vi "Nicmos_Test.vi"() -> ()   [LabVIEW 2009]
uses:
  Controls/NICMOS.READOUT.ctl
  <vilib>/Analysis/2dsp.llb/Power Spectrum (DBL).vi
  <vilib>/Analysis/NI_AALBase.lvlib
  <vilib>/Analysis/NI_AALPro.lvlib
panel:
  in  "READOUT":T1={"Readout"=8, "Deglitch"=2, "Framerate"=40.061293779482604, "Bank"=6}
  in  "Commande onglet":T2(tab)=enum."Zoom"
  out "Std Dev 2":dbl=47.642857142857146 format="%.1f"
  out "Std Dev":dbl=6.902380541730306 format="%.1f"
  in  "Integrate pattern":bool
  out "Mean Level":dbl=112.25 format="%.1f"
  out "Total NRJ":i32=11694532
  out "Scan":i32[](graph)=[115, 117, 121, 110, 109, 113, 115, 98]
  out "Image":i32[][](graph)
  out "Power Spectrum":cluster{dbl[unit][], "Power Spectrum":dbl[]}(graph)={[0.0, 5.7230419684975145, 11.446083936995029, 17.169125905492542, 22.892167873990058, 28.615209842487573, 34.338251810985085, 40.0612937794826], "Power Spectrum"=[12600.0625, 4.685660171779821, 9.8125, 2.5643398282201786, 7.5625, 2.5643398282201786, 9.8125, 4.685660171779821]}
  out "y":dbl=39.77045768581225 format="%.1f"
  out "x":dbl=48.747249279268516 format="%.1f"
  out "b":dbl=0.5346203674875701 format="%.2f"
  out "theta":dbl[unit]=0.3638978669091496 format="%.2f"
  out "a":dbl=0.46263779966875623 format="%.2f"
  out "Graphe d'intensité 2":i32[][](graph)
  out "Y":dbl=40.58244294659929 format="%.2f"
  out "X":dbl=36.54206833038434 format="%.2f"
  out "Waist  Y":dbl=7.63982963428037 format="%.2f"
  out "Waist  X":dbl=1.8793090656266391 format="%.2f"
  out "Cut X":i32[](graph)=[103, 83, 96, 100, 88, 113, 103, 107, 94, 113, 101, 105, 126, 101, 82, 109, 104, 107, 107, 108, 103, 108, 108, 95, 109, 125, 112, 101, 110, 121, 107, 114, 120, 130, 485, 4787, 15469, 16134, 5594, 626, 166, 133, 128, 97, 117, 107, 102, 100, 95, 95, 106, 96, 97, 116, 98, 98, 101, 87, 90, 102, 106, 118, 93, 82, 102, 84, 92, 86, 107, 93, 102, 90, 95, 111, 84, 90, 100, 91, 99, 88, 76, 95, 86, 95, 99, 106, 91, 84, 106, 92, 89, 94, 85, 102, 80, 105, 102, 92, 94, 94]
  out "Cut Y":i32[](graph)=[120, 126, 140, 107, 115, 124, 117, 130, 100, 122, 124, 123, 118, 134, 131, 129, 116, 118, 141, 134, 132, 157, 120, 159, 184, 212, 298, 440, 547, 793, 1032, 1285, 1844, 2542, 3680, 5646, 7465, 9888, 12467, 13747, 15731, 16134, 14689, 11843, 10941, 8277, 6077, 3654, 2326, 1431, 770, 403, 229, 155, 127, 127, 120, 135, 110, 111, 129, 123, 107, 139, 134, 127, 146, 219, 255, 385, 410, 516, 696, 659, 728, 697, 619, 481, 433, 338, 246, 203, 160, 136, 134, 129, 119, 114, 89, 120, 96, 101, 6, 116, 102, 105, 8, 95, 112, 95]
  out "TF":dbl[](graph)=[45.4276, 21.636402236844145, 4.179884490958335, 2.464480404857662, 1.825830498475382, 0.8054648624902895, 2.1657476536706626, 4.800193289283871, 6.927657461153612, 0.07664838527835617, 0.22072977933809118, 0.3119619762944224, 1.342643246229423, 1.308546944749124, 1.7136756152866615, 3.5009415033794906, 0.7351378410487727, 3.8469382391196723, 2.278880052659914, 1.922968432633993, 5.308677333059524, 3.359421176595885, 6.962587944848487, 0.3974776855929291, 0.3142220112327611, 3.7, 0.5645988968260751, 2.396325978160049, 2.9447944036965015, 0.41922086515161655, 2.1562702206619084, 4.50890531491479, 7.49681636589277, 1.3066799564956808, 1.505991764306582, 0.8319064647461071, 1.3923532021524945, 5.642854556851627, 0.38294572116738607, 2.3154461070592256, 0.510522666940476, 1.1264207963434756, 0.2861216373661286, 2.5174300191340806, 0.69422487709815, 0.292687169384113, 0.1900662229097688, 3.776102968784432, 0.7608200930201349, 0.9345746658549572, 2.25, 0.9345746658549572, 0.7608200930201349, 3.776102968784432, 0.1900662229097688, 0.292687169384113, 0.69422487709815, 2.5174300191340806, 0.2861216373661286, 1.1264207963434756, 0.510522666940476, 2.3154461070592256, 0.38294572116738607, 5.642854556851627, 1.3923532021524945, 0.8319064647461071, 1.505991764306582, 1.3066799564956808, 7.49681636589277, 4.50890531491479, 2.1562702206619084, 0.41922086515161655, 2.9447944036965015, 2.396325978160049, 0.5645988968260751, 3.7, 0.3142220112327611, 0.3974776855929291, 6.962587944848487, 3.359421176595885, 5.308677333059524, 1.922968432633993, 2.278880052659914, 3.8469382391196723, 0.7351378410487727, 3.5009415033794906, 1.7136756152866615, 1.308546944749124, 1.342643246229423, 0.3119619762944224, 0.22072977933809118, 0.07664838527835617, 6.927657461153612, 4.800193289283871, 2.1657476536706626, 0.8054648624902895, 1.825830498475382, 2.464480404857662, 4.179884490958335, 21.636402236844145]
  out "Vertical cut":dbl[](graph)=[30.0, 15.0, 24.0, 32.0, 17.0, 10.0, 18.0, 4.0, 15.0, 9.0, -10.0, 25.0, 20.0, 22.0, 17.0, 2.0, 13.0, 18.0, -14.0, 10.0, -2.0, -8.0, -8.0, -5.0, 5.0, -14.0, 2.0, 10.0, -4.0, -20.0, 6.0, 5.0, 2.0, -8.0, -9.0, -6.0, -6.0, -19.0, 9.0, 4.0, 1.0, -6.0, 6.0, -2.0, -8.0, -1.0, -3.0, 21.0, 13.0, 8.0, -5.0, 5.0, 13.0, 10.0, -14.0, -3.0, -1.0, 3.0, 11.0, 1.0, 15.0, 23.0, 11.0, -3.0, -2.0, -3.0, 9.0, 21.0, 6.0, -103.0, 5.0, 19.0, 8.0, 13.0, 15.0, 4.0, 21.0, 28.0, 12.0, 13.0, 25.0, 15.0, 9.0, 11.0, 20.0, -2.0, 19.0, 22.0, 17.0, 37.0, 25.0, 0.0, 14.0, 15.0, 9.0, 14.0, 15.0, 2.0, 21.0, 14.0]
  out "DSP":cluster{dbl[unit][], "Power Spectrum":dbl[]}(graph)={[0.0, 5.7230419684975145, 11.446083936995029, 17.169125905492542, 22.892167873990058, 28.615209842487573, 34.338251810985085, 40.0612937794826], "Power Spectrum"=[]}
  in  "RESET ACCUMULATE":bool
  in  "RESET ACCUMULATE 2":bool
  out "Graphe XY":cluster{dbl[], dbl[]}(graph)={[1341175.125, 1343537.125, 1345374.5, 1349276.0, 1353395.625, 1355804.625, 1356299.25, 1315217.375, 1314825.25], [2425317.4836309524, 2730754.322916748, 3781664.8095238847, 1635464.059523804, 5468045.299107264, 1983356.644345304, 2776568.125, 1310442574.483631, 1184346966.910715]}
  out "Standard Deviation":dbl(graph)=100014.63289358855
  in  "Filter?":bool
  out "Graphe XY 2":cluster{dbl[unit][], "Power Spectrum":dbl[]}(graph)={[0.0, 5.7230419684975145, 11.446083936995029, 17.169125905492542, 22.892167873990058, 28.615209842487573, 34.338251810985085, 40.0612937794826], "Power Spectrum"=[1732307746455.1406, 2670579822.32282, 1023845913.265625, 501399858.4584302, 360909755.640625, 501399858.4584302, 1023845913.265625, 2670579822.32282]}
  out "Graphe":dbl[](graph)=[1505710.0, 1422929.0, 1333372.0, 1291362.0, 1266016.0, 1249535.0, 1235579.0, 1224870.0]
  in  "Freq":dbl[](array[numeric])
  out "Time":dbl[unit]=2.4961750000000003e-06
  out "Graphe 2":i32[](graph)
  in  "UPDATE":bool
  in  "Image index":i32
  in  "STOP":bool
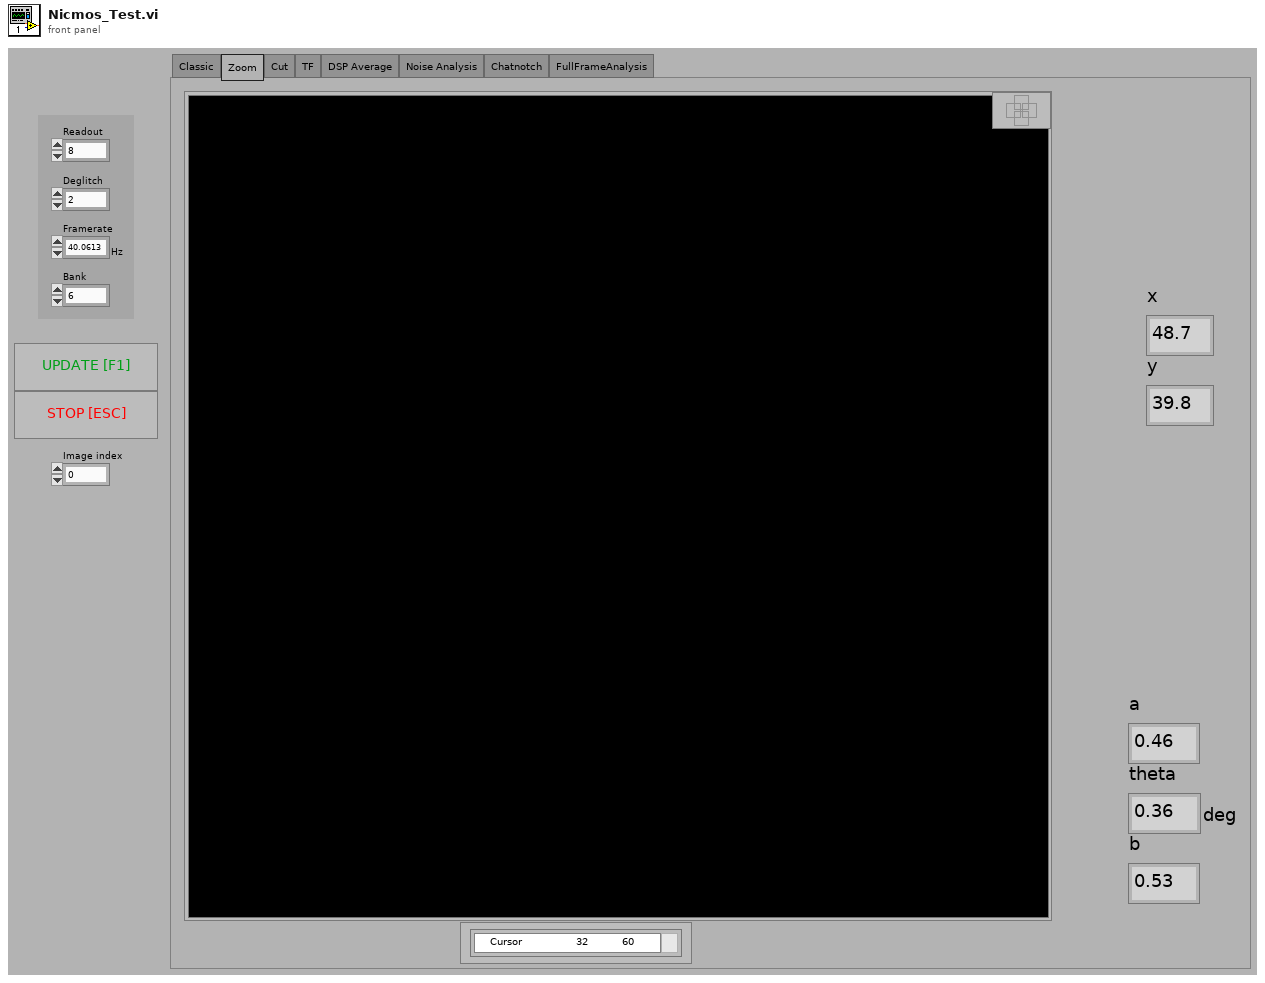
[diagram p1: front panel]
types:
  T1 = typedef "NICMOS.READOUT.ctl" = cluster{"Readout":i32, "Deglitch":i32, "Framerate":dbl[unit], "Bank":i32}
  T2 = enum32{"Classic", "Zoom", "Cut", "TF", "DSP Average", "Noise Analysis", "Chatnotch", "FullFrameAnalysis"}
  T3 = typedef "NICMOS.DATA.ctl" = cluster{"DATA":i32[][][], "INDEX":i32}
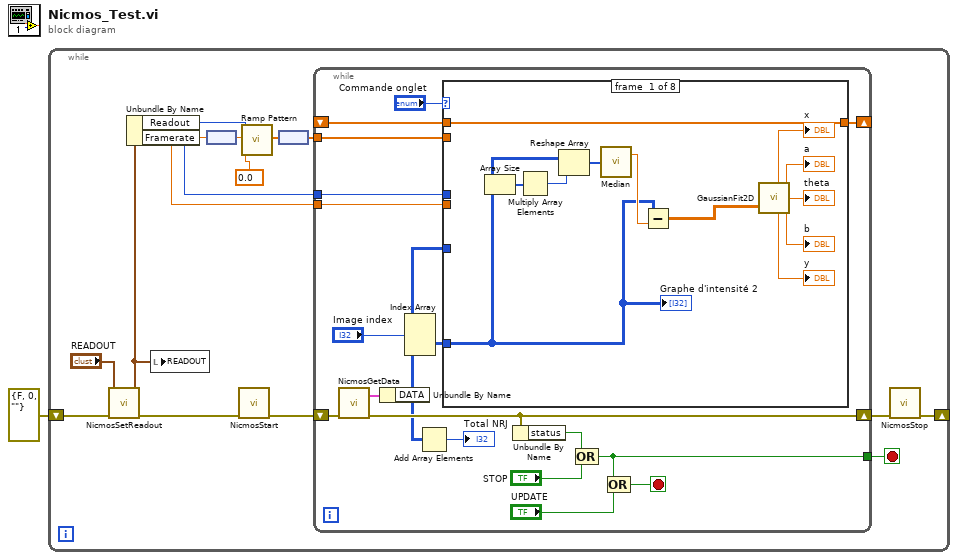
[diagram p0: block diagram]
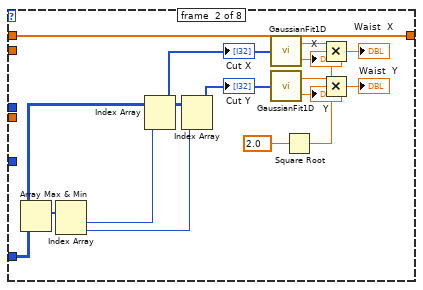
[diagram p2: hidden frame]
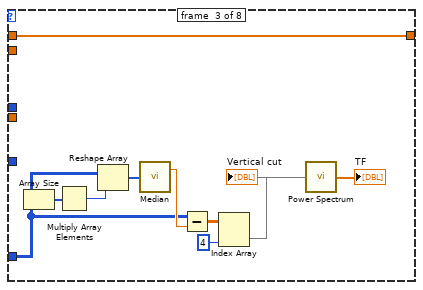
[diagram p3: hidden frame]
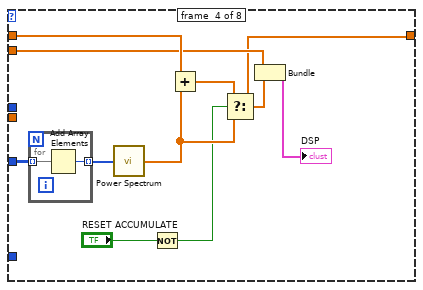
[diagram p4: hidden frame]
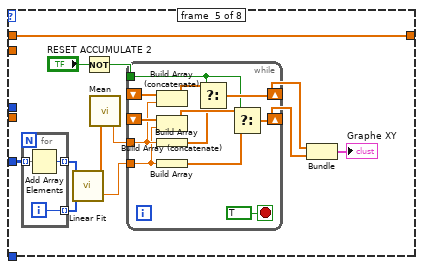
[diagram p5: hidden frame]
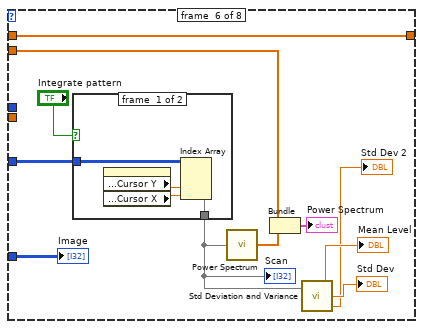
[diagram p6: hidden frame]
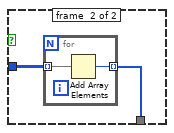
[diagram p7: hidden frame]
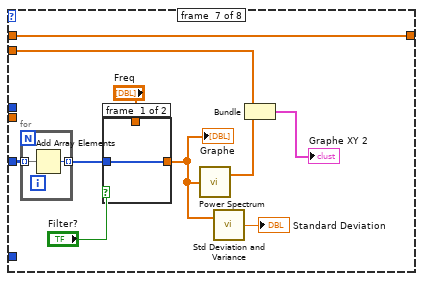
[diagram p8: hidden frame]
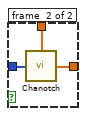
[diagram p9: hidden frame]
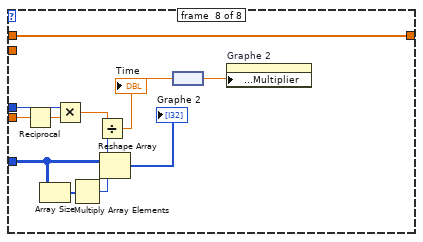
[diagram p10: hidden frame]
diagram:
  n1 = while {
    shift-right: [w6] -> _
    shift-left: errorcluster {"status"=FALSE, "code"=0, "source"=""} ("error out") -> [w15]
    stop <- w14 stop-if-true
    n2 = call "NicmosSetReadout.vi"("READOUT in"="READOUT", "error in (no error)"=w15) -> ("READOUT out"=w4:T1, "error out"=w9:errorcluster)  [unwired: 6 in]
    n3 = Unbundle By Name(w4) -> ("Readout"=w2:i32, "Framerate"=w3:dbl[unit])
    n4 = local write "READOUT"(w4) -> ()
    n5 = node(w3) -> (w12:dbl)
    n6 = call "NicmosStart.vi"("error in (no error)"=w9) -> ("error out"=w8:errorcluster)  [unwired: 8 in]
    n7 = call <vilib>:"Ramp Pattern.vi"("start"=0.0, "end"=w12, "samples"=w2) -> ("Ramp Pattern"=w11:dbl[])  [unwired: 7 in, 1 out]
    n8 = node(w11) -> (w10:dbl[unit][])
    n9 = while {
      shift-left: w8 -> [w23]
      shift-right: [w22] -> w7
      tunnel: [w29] -> w14
      tunnel: w10 -> [w28]
      shift-right: [w20] -> _
      shift-left: _ -> [w21]
      tunnel: w3 -> [w19]
      tunnel: w2 -> [w18]
      stop <- w30 stop-if-true
      n10 = call "NicmosGetData.vi"("error in (no error)"=w23) -> ("DATA"=w17:T3, "error out"=w22:errorcluster)  [unwired: 7 in]
      n11 = Unbundle By Name(w17) -> ("DATA"=w16:i32[][][])
      n12 = Index Array(array=w16, index (dim 0)="Image index") -> (element=w27:i32[][])  [unwired: 2 in]
      n13 = Add Array Elements(numeric array=w16) -> (sum=→"Total NRJ":i32)
      n14 = case shown="\"FullFrameAnalysis\"" "Commande onglet" {
        tunnel: w28 -> [_ _ _ w73 _ w120 w134 _]
        tunnel: w27 -> [w35 w47 w66 _ _ w117 _ _]
        tunnel: w16 -> [_ _ _ w80 w90 w115 w138 w154]
        tunnel: w21 -> [w34 w46 w61 w78 w94 w111 w135 w153]
        tunnel: [w34 w46 w61 w72 w94 w111 w135 w153] -> w20
        tunnel: w19 -> [_ _ _ _ _ _ _ w152]
        tunnel: w18 -> [_ _ _ _ _ _ _ w151]
        frame #0 {
          n15 = Array Size(array=w35) -> (size(s)=w44:i32[])
          n16 = Multiply Array Elements(1:w44) -> (0:w43:i32)
          n17 = Reshape Array(w35, w43) -> (w42:i32[])
          n18 = call <vilib>:"Median.vi"("X"=w42) -> ("median"=w40:dbl)  [unwired: 1 out]
          n19 = Subtract(x=w35, y=w40) -> (x-y=w41:dbl[][])
          n20 = call "GaussianFit2D.vi"("Image"=w41) -> ("b"=→"b":dbl, "y"=→"y":dbl, "theta"=→"theta":dbl[unit], "a"=→"a":dbl, "x"=→"x":dbl)  [unwired: 1 in]
          "Graphe d'intensité 2" <- w35
        }
        frame #1 {
          n21 = Array Max & Min(array=w47) -> (max index (indices)=w60:i32[])  [unwired: 3 out]
          n22 = Index Array(array=w60) -> (element #1=w57:i32, element #2=w58:i32)  [unwired: 2 in]
          n23 = Index Array(array=w47, index (row)=w57) -> (element=w59:i32[])  [unwired: 1 in]
          "Cut X" <- w59
          n24 = Index Array(array=w47, index (col)=w58) -> (element=w56:i32[])  [unwired: 1 in]
          "Cut Y" <- w56
          n25 = call "GaussianFit1D.vi"("Cut"=w59) -> ("Sigma"=w55:dbl, "x"=→"X":dbl)
          n26 = call "GaussianFit1D.vi"("Cut"=w56) -> ("Sigma"=w54:dbl, "x"=→"Y":dbl)
          n27 = Square Root(x=2.0) -> (sqrt(x)=w51:dbl)
          n28 = Multiply(x=w55, y=w51) -> (x*y=→"Waist  X":dbl)
          n29 = Multiply(x=w54, y=w51) -> (x*y=→"Waist  Y":dbl)
        }
        frame #2 {
          n30 = Array Size(array=w66) -> (size(s)=w70:i32[])
          n31 = Multiply Array Elements(1:w70) -> (0:w69:i32)
          n32 = Reshape Array(w66, w69) -> (w68:i32[])
          n33 = call <vilib>:"Median.vi"("X"=w68) -> ("median"=w67:dbl)  [unwired: 1 out]
          n34 = Subtract(x=w66, y=w67) -> (x-y=w65:dbl[][])
          n35 = Index Array(array=w65, index (col)=4 ("indice désactivé (col)")) -> (element=w63:dbl[])  [unwired: 1 in]
          "Vertical cut" <- w63
          n36 = call-poly <vilib>:"Power Spectrum.vi"("X"=w63) -> ("Power Spectrum"=→"TF":dbl[])  [unwired: 1 out]
        }
        frame #3 {
          n37 = for {
            tunnel: w80 -> [w82] mode=indexing
            tunnel: [w81] -> w79 mode=indexing
            n38 = Add Array Elements(numeric array=w82) -> (sum=w81:i32)
          }
          n39 = call-poly <vilib>:"Power Spectrum.vi"("X"=w79) -> ("Power Spectrum"=w76:dbl[])  [unwired: 1 out]
          n40 = Not(x="RESET ACCUMULATE") -> (.not. x?=w74:bool)
          n41 = Add(x=w78, y=w76) -> (x+y=w75:dbl[])
          n42 = Select(t=w75, s=w74, f=w76) -> (s? t:f=w72:dbl[])
          n43 = Bundle(w73, "Power Spectrum"=w72) -> (→"DSP":cluster{dbl[unit][], "Power Spectrum":dbl[]})  [unwired: 1 in]
        }
        frame #4 {
          n44 = for {
            tunnel: w90 -> [w109] mode=indexing
            tunnel: [w108] -> w86 mode=indexing
            tunnel: [w107] -> w87 mode=indexing
            i -> [w107]
            n45 = Add Array Elements(numeric array=w109) -> (sum=w108:i32)
          }
          n46 = call <vilib>:"Linear Fit.vi"("Y"=w86, "X"=w87) -> ("Best Linear Fit"=w84:dbl[], "residue"=w85:dbl)  [unwired: 9 in, 3 out]
          n47 = Not(x="RESET ACCUMULATE 2") -> (.not. x?=w88:bool)
          n48 = call <vilib>:"Mean.vi"("X"=w84) -> ("mean"=w83:dbl)  [unwired: 1 out]
          n49 = while {
            tunnel: w83 -> [w98]
            tunnel: w85 -> [w97]
            shift-right: [w104] -> w92
            shift-left: _ -> [w105]
            shift-right: [w102] -> w93
            shift-left: _ -> [w103]
            tunnel: w88 -> [w101]
            stop <- TRUE stop-if-true
            n50 = Build Array (concatenate)(w105, w98) -> (w100:dbl[])
            n51 = Build Array (concatenate)(w103, w97) -> (w99:dbl[])
            n52 = Build Array(w98) -> (w96:dbl[])
            n53 = Build Array(w97) -> (w95:dbl[])
            n54 = Select(t=w100, s=w101, f=w96) -> (s? t:f=w104:dbl[])
            n55 = Select(t=w99, s=w101, f=w95) -> (s? t:f=w102:dbl[])
          }
          n56 = Bundle(w92, w93) -> (→"Graphe XY":cluster{dbl[], dbl[]})  [unwired: 1 in]
        }
        frame #5 {
          n57 = case shown="True" "Integrate pattern" {
            tunnel: w115 -> [w123 w126]
            tunnel: [w122 w125] -> w114
            frame #0 {
              n58 = property on="Image" class="GraphIntens (strict)"() -> ("Cursor.Cursor Position:Cursor Y"=w124:dbl, "Cursor.Cursor Position:Cursor X"=w121:dbl)  [unwired: 2 in, 2 out]
              n59 = Index Array(array=w123, index (dim 1)=w124, index (dim 2)=w121) -> (element=w122:i32[])  [unwired: 1 in]
            }
            frame #1 {
              n60 = for {
                tunnel: w126 -> [w128] mode=indexing
                tunnel: [w127] -> w125 mode=indexing
                n61 = Add Array Elements(numeric array=w128) -> (sum=w127:i32)
              }
            }
          }
          "Scan" <- w114
          n62 = call-poly <vilib>:"Power Spectrum.vi"("X"=w114) -> ("Power Spectrum"=w118:dbl[])  [unwired: 1 out]
          n63 = Bundle(w120, "Power Spectrum"=w118) -> (→"Power Spectrum":cluster{dbl[unit][], "Power Spectrum":dbl[]})  [unwired: 1 in]
          n64 = call <vilib>:"Std Deviation and Variance.vi"("X"=w114) -> ("mean"=→"Mean Level":dbl, "standard deviation"=→"Std Dev":dbl, "variance"=→"Std Dev 2":dbl)  [unwired: 1 in]
          "Image" <- w117
        }
        frame #6 {
          n65 = for {
            tunnel: w138 -> [w144] mode=indexing
            tunnel: [w143] -> w137 mode=indexing
            n66 = Add Array Elements(numeric array=w144) -> (sum=w143:i32)
          }
          n67 = case shown="False" "Filter?" {
            tunnel: w137 -> [w139 w142]
            tunnel: "Freq" -> [_ w141]
            tunnel: [w139 w140] -> w130
            frame #0 {
            }
            frame #1 {
              n68 = call "Chanotch.vi"("Signal"=w142, "Freq"=w141) -> ("Chanotched Signal"=w140:dbl[])
            }
          }
          "Graphe" <- w130
          n69 = call-poly <vilib>:"Power Spectrum.vi"("X"=w130) -> ("Power Spectrum"=w133:dbl[])  [unwired: 1 out]
          n70 = call <vilib>:"Std Deviation and Variance.vi"("X"=w130) -> ("standard deviation"=→"Standard Deviation":dbl)  [unwired: 1 in, 2 out]
          n71 = Bundle(w134, "Power Spectrum"=w133) -> (→"Graphe XY 2":cluster{dbl[unit][], "Power Spectrum":dbl[]})  [unwired: 1 in]
        }
        frame #7 {
          n72 = Reciprocal(x=w152) -> (1/x=w150:dbl[unit])
          n73 = Array Size(array=w154) -> (size(s)=w155:i32[])
          n74 = Multiply(x=w151, y=w150) -> (x*y=w148:dbl[unit])
          n75 = Multiply Array Elements(1:w155) -> (0:w147:i32)
          n76 = Divide(x=w148, y=w147) -> (x/y=w146:dbl[unit])
          "Time" <- w146
          n77 = Reshape Array(w154, w147) -> (→"Graphe 2":i32[])
          n78 = node(w146) -> (w145:dbl)
          n79 = property on="Graphe 2" class="GrapheWaveform (strict)"("X Scale.Offset and Multiplier:Multiplier"=w145) -> ()  [unwired: 2 in, 2 out]
        }
      }
      n80 = Unbundle By Name(w22) -> ("status"=w33:bool)
      n81 = Compound Arithmetic op=OR(w33, "STOP") -> (w29:bool)
      n82 = Compound Arithmetic op=OR(w29, "UPDATE") -> (w30:bool)
    }
    n83 = call "NicmosStop.vi"("error in (no error)"=w7) -> ("error out"=w6:errorcluster)  [unwired: 8 in]
  }
